vi "REPORT_AUDIT_rows_style_pdf.vi"(11 "REPORT_AUDIT_all_info":T1) -> (3 "Row  [ ]":T3)   [LabVIEW 2020]
uses:
  <vilib>/Exaprom PDF/Controls/Table Controls/Table Appearance and Font Row [ ].ctl
  <vilib>/Exaprom PDF/Controls/Table Controls/One Row Appearance.ctl
  <vilib>/Exaprom PDF/Controls/Table Controls/Row from to.ctl
  <vilib>/Exaprom PDF/Controls/Table Controls/Cell, Alignment, LS and Font - hide Vmerge.ctl
  <vilib>/Exaprom PDF/Controls/Table Controls/Cell Type, Alignment and LS.ctl
  <vilib>/Exaprom PDF/Controls/Table Controls/Cell Alignment 20px.ctl
  <vilib>/Exaprom PDF/Controls/Table Controls/Text vertical arrangement.ctl
  <vilib>/Exaprom PDF/Controls/Text Controls/Line spacing.ctl
  <vilib>/Exaprom PDF/Controls/Table Controls/Cell Appearance.ctl
  <vilib>/Exaprom PDF/Controls/Table Controls/Cell Border 20 px.ctl
  <vilib>/Exaprom PDF/Controls/Table Controls/Merge Horizontal.ctl
  <vilib>/Exaprom PDF/Controls/Table Controls/Merge Vertical.ctl
  <vilib>/Exaprom PDF/Controls/Font Controls/Font complete cluster.ctl
  <vilib>/Exaprom PDF/Controls/Font Controls/Font size.ctl
  <vilib>/Exaprom PDF/Controls/Font Controls/Font color.ctl
  <vilib>/Exaprom PDF/Controls/Font Controls/Type and encoding.ctl
  <vilib>/Exaprom PDF/Controls/Text Controls/Unicode/Type and run direction.ctl
  typedef/REPORT_AUDIT_all_info.ctl
  GEAR/typedef/REPORT_GEAR_statuses.ctl
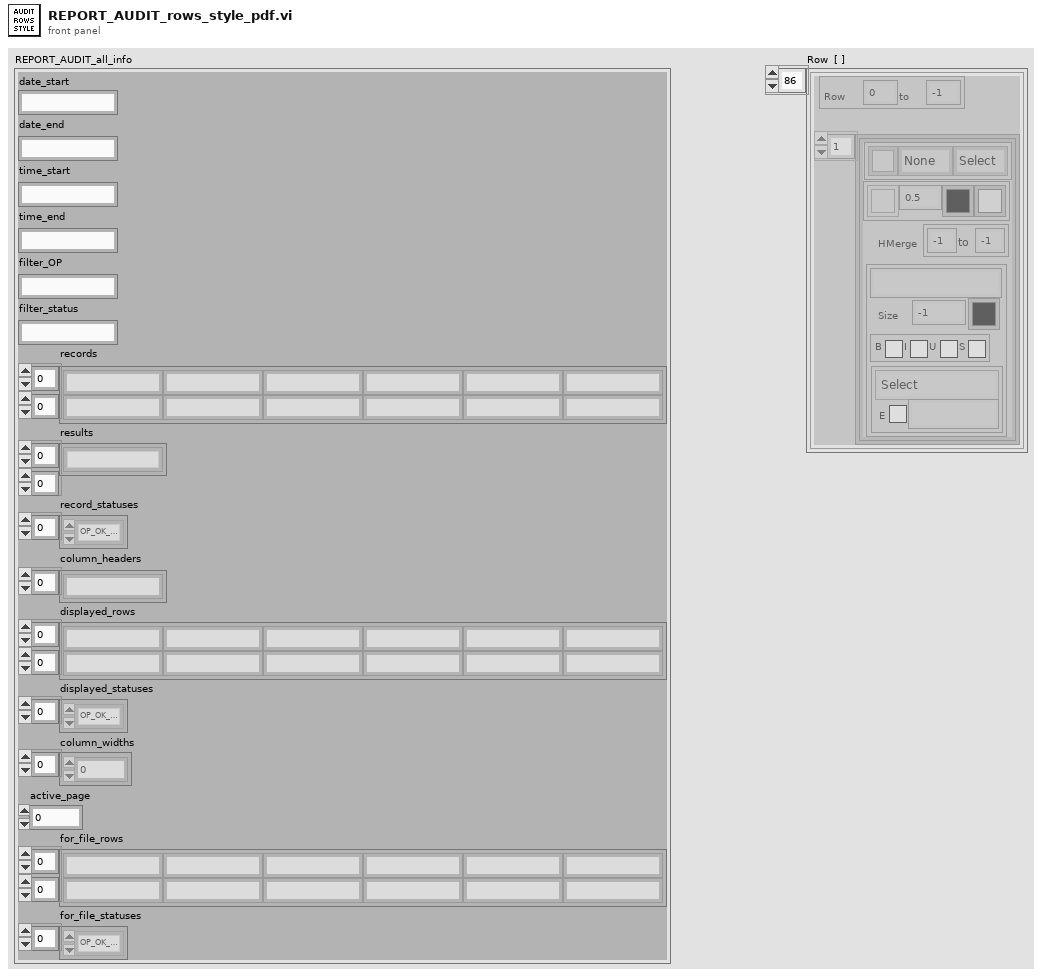
[diagram p1: front panel]
types:
  T1 = typedef "REPORT_AUDIT_all_info.ctl" = cluster{"date_start":string, "date_end":string, "time_start":string, "time_end":string, "filter_OP":string, "filter_status":string, "records":string[][], "results":string[][], "record_statuses":T2[], "column_headers":string[], "displayed_rows":string[][], "displayed_statuses":T2[], "column_widths":i16[], "active_page":i32, "for_file_rows":string[][], "for_file_statuses":T2[]}
  T2 = typedef "REPORT_GEAR_statuses.ctl" = enum16{"OP_OK_hide", "OP_OK_show", "OP_NOK_hide", "OP_NOK_show", "OP_interrupted_hide", "OP_interrupted_show", "OP_in_operation_hide", "OP_in_operation_show", "OP_unexpected_hide", "OP_unexpected_show", "RE_REAL_OK", "RE_REAL_NOK", "RE_STRING", "RE_sub_header", "RE_no_data", "RE_unexpected", "BA_sub_header", "BA_data", "BA_no_data"}
  T3 = typedef "Table Appearance and Font Row [ ].ctl" = T4[]
  T4 = typedef "One Row Appearance.ctl" = cluster{"Row":T5, "Cell [ ]":T6[]}
  T5 = typedef "Row from to.ctl" = cluster{"From #":i16, "to #":i16}
  T6 = typedef "Cell, Alignment, LS and Font - hide Vmerge.ctl" = cluster{"Text":T7, "Cell Appearance":T11, "HMerge":T13, "VMerge":T14, "Font":T15}
  T7 = typedef "Cell Type, Alignment and LS.ctl" = cluster{"Cell Alignment":T8, "Text rotation":T9, "Line spacing":T10}
  T8 = typedef "Cell Alignment 20px.ctl" = u16
  T9 = typedef "Text vertical arrangement.ctl" = enum16{"None", "Clockwise", "Counterclockwise"}
  T10 = typedef "Line spacing.ctl" = enum16{"Select", "1.0", "1.5", "2.0"}
  T11 = typedef "Cell Appearance.ctl" = cluster{"Border":T12, "Thickness":sgl, "Color":u32, "BG":u32}
  T12 = typedef "Cell Border 20 px.ctl" = u16
  T13 = typedef "Merge Horizontal.ctl" = cluster{"From":i8, "to":i8}
  T14 = typedef "Merge Vertical.ctl" = cluster{"From":i8, "to":i8}
  T15 = typedef "Font complete cluster.ctl" = cluster{"Name":string, "Size":T16, "Color":T17, "Style":cluster{"Bold":bool, "Italic":bool, "Underline":bool, "Strikeout":bool}, "Type":T18}
  T16 = typedef "Font size.ctl" = sgl
  T17 = typedef "Font color.ctl" = u32
  T18 = typedef "Type and encoding.ctl" = cluster{"Type&direction":T19, "Embedded":bool, "Encoding":string}
  T19 = typedef "Type and run direction.ctl" = enum16{"Select", "ASCII", "UTF-16", "UTF-16 (default)", "UTF-16 (LTR)", "UTF-16 (RTL)"}
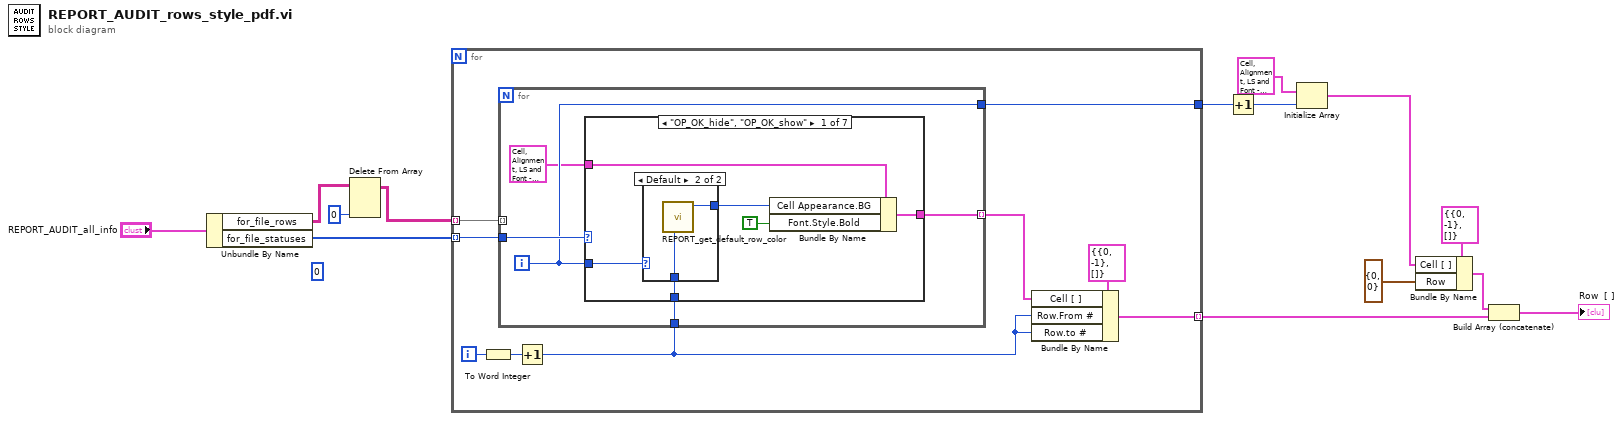
[diagram p0: block diagram]
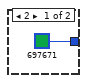
[diagram p2: hidden frame]
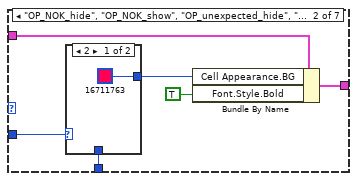
[diagram p3: hidden frame]
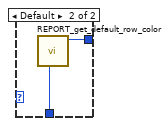
[diagram p4: hidden frame]
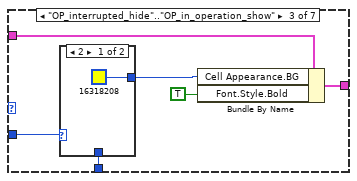
[diagram p5: hidden frame]
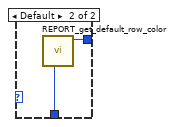
[diagram p6: hidden frame]
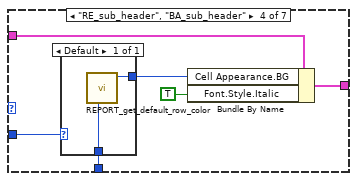
[diagram p7: hidden frame]
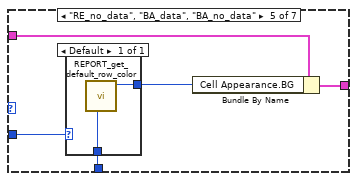
[diagram p8: hidden frame]
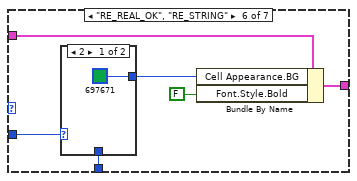
[diagram p9: hidden frame]
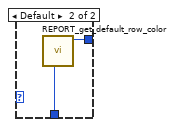
[diagram p10: hidden frame]
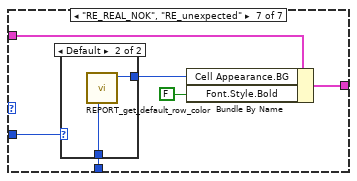
[diagram p11: hidden frame]
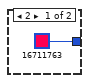
[diagram p12: hidden frame]
diagram:
  (unwired) 0
  n1 = Unbundle By Name("REPORT_AUDIT_all_info") -> ("for_file_rows"=w4:string[][], "for_file_statuses"=w1:T2[])
  n2 = Delete From Array(array=w4, index (col)=0) -> (array with subset deleted=w2:string[][])  [unwired: 2 in, 1 out]
  n3 = for {
    tunnel: w2 -> [w19] mode=indexing
    tunnel: w1 -> [w18] mode=indexing
    tunnel: [w22] -> w12 mode=indexing
    tunnel: [w15] -> w6
    i -> [w21]
    n4 = To Word Integer(number=w21) -> (16bit integer=w20:i16)
    n5 = Increment(x=w20) -> (x+1=w16:i16)
    n6 = for {
      tunnel: w19 -> [_] mode=indexing
      tunnel: w18 -> [w28]
      tunnel: [w27] -> w17 mode=indexing
      tunnel: w16 -> [w24]
      tunnel: [w26] -> w15
      i -> [w26]
      n7 = case shown="\"OP_OK_hide\", \"OP_OK_show\"" w28 {
        tunnel: T6 {"Text"={"Cell Alignment"=0, "Text rotation"=enum."None", "Line spacing"=enum."Select"}, "Cell Appearance"={"Border"=5, "Thickness"=0.5, "Color"=0, "BG"=16448250}, "HMerge"={"From"=-1, "to"=-1}, "VMerge"={"From"=-1, "to"=-1}, "Font"={"Name"="Consolas", "Size"=10.0, "Color"=0, "Style"={"Bold"=FALSE, "Italic"=FALSE, "Underline"=FALSE, "Strikeout"=FALSE}, "Type"={"Type&direction"=enum."ASCII", "Embedded"=FALSE, "Encoding"="CP855"}}} ("Cell, Alignment, LS and Font") -> [w34 w41 w50 w59 w66 w73 w82]
        tunnel: [w31 w40 w47 w58 w67 w74 w83] -> w27
        tunnel: w26 -> [w30 w39 w49 w56 w65 w72 w81]
        tunnel: w24 -> [w29 w38 w48 w57 w64 w71 w80]
        frame "OP_OK_hide", "OP_OK_show" {
          n8 = case shown="Default" w30 {
            tunnel: [u32 697671 w37] -> w32
            tunnel: w29 -> [_ w36]
            frame 2 {
            }
            frame Default {
              n9 = call "REPORT_get_default_row_color.vi"("row"=w36) -> ("color"=w37:u32)  [unwired: 10 in]
            }
          }
          n10 = Bundle By Name(cluster=w34, "Cell Appearance.BG"=w32, "Font.Style.Bold"=TRUE ("Active Cell:Cell Font:Bold")) -> (w31:T6)
        }
        frame "OP_NOK_hide", "OP_NOK_show", "OP_unexpected_hide", "OP_unexpected_show" {
          n11 = case shown="2" w39 {
            tunnel: [u32 16711763 w46] -> w42
            tunnel: w38 -> [_ w45]
            frame 2 {
            }
            frame Default {
              n12 = call "REPORT_get_default_row_color.vi"("row"=w45) -> ("color"=w46:u32)  [unwired: 10 in]
            }
          }
          n13 = Bundle By Name(cluster=w41, "Cell Appearance.BG"=w42, "Font.Style.Bold"=TRUE ("Active Cell:Cell Font:Bold")) -> (w40:T6)
        }
        frame "OP_interrupted_hide".."OP_in_operation_show" {
          n14 = case shown="2" w49 {
            tunnel: [u32 16318208 w55] -> w52
            tunnel: w48 -> [_ w54]
            frame 2 {
            }
            frame Default {
              n15 = call "REPORT_get_default_row_color.vi"("row"=w54) -> ("color"=w55:u32)  [unwired: 10 in]
            }
          }
          n16 = Bundle By Name(cluster=w50, "Cell Appearance.BG"=w52, "Font.Style.Bold"=TRUE ("Active Cell:Cell Font:Bold")) -> (w47:T6)
        }
        frame "RE_sub_header", "BA_sub_header" {
          n17 = case shown="Default" w56 {
            tunnel: [w63] -> w61
            tunnel: w57 -> [w62]
            frame Default {
              n18 = call "REPORT_get_default_row_color.vi"("row"=w62) -> ("color"=w63:u32)  [unwired: 10 in]
            }
          }
          n19 = Bundle By Name(cluster=w59, "Cell Appearance.BG"=w61, "Font.Style.Italic"=TRUE ("Active Cell:Cell Font:Bold")) -> (w58:T6)
        }
        frame "RE_no_data", "BA_data", "BA_no_data" {
          n20 = case shown="Default" w65 {
            tunnel: [w70] -> w68
            tunnel: w64 -> [w69]
            frame Default {
              n21 = call "REPORT_get_default_row_color.vi"("row"=w69) -> ("color"=w70:u32)  [unwired: 10 in]
            }
          }
          n22 = Bundle By Name(cluster=w66, "Cell Appearance.BG"=w68) -> (w67:T6)
        }
        frame "RE_REAL_OK", "RE_STRING" {
          n23 = case shown="2" w72 {
            tunnel: [u32 697671 w79] -> w76
            tunnel: w71 -> [_ w78]
            frame 2 {
            }
            frame Default {
              n24 = call "REPORT_get_default_row_color.vi"("row"=w78) -> ("color"=w79:u32)  [unwired: 10 in]
            }
          }
          n25 = Bundle By Name(cluster=w73, "Cell Appearance.BG"=w76, "Font.Style.Bold"=FALSE ("Active Cell:Cell Font:Bold")) -> (w74:T6)
        }
        frame "RE_REAL_NOK", "RE_unexpected" {
          n26 = case shown="Default" w81 {
            tunnel: [u32 16711763 w88] -> w85
            tunnel: w80 -> [_ w87]
            frame 2 {
            }
            frame Default {
              n27 = call "REPORT_get_default_row_color.vi"("row"=w87) -> ("color"=w88:u32)  [unwired: 10 in]
            }
          }
          n28 = Bundle By Name(cluster=w82, "Cell Appearance.BG"=w85, "Font.Style.Bold"=FALSE ("Active Cell:Cell Font:Bold")) -> (w83:T6)
        }
      }
    }
    n29 = Bundle By Name(cluster=T4 {"Row"={"From #"=0, "to #"=-1}, "Cell [ ]"=[]} ("Row Appearance and Font  [ ]"), "Cell [ ]"=w17, "Row.From #"=w16, "Row.to #"=w16) -> (w22:T4)
  }
  n30 = Increment(x=w6) -> (x+1=w5:i32)
  n31 = Initialize Array(T6 {"Text"={"Cell Alignment"=0, "Text rotation"=enum."None", "Line spacing"=enum."Select"}, "Cell Appearance"={"Border"=5, "Thickness"=1.5, "Color"=16777228, "BG"=16448250}, "HMerge"={"From"=-1, "to"=-1}, "VMerge"={"From"=-1, "to"=-1}, "Font"={"Name"="Consolas", "Size"=10.0, "Color"=16777228, "Style"={"Bold"=TRUE, "Italic"=FALSE, "Underline"=FALSE, "Strikeout"=FALSE}, "Type"={"Type&direction"=enum."ASCII", "Embedded"=FALSE, "Encoding"="CP855"}}} ("Cell, Alignment, LS and Font"), w5) -> (w8:T6[])
  n32 = Bundle By Name(cluster=T4 {"Row"={"From #"=0, "to #"=-1}, "Cell [ ]"=[]} ("Row Appearance and Font  [ ]"), "Cell [ ]"=w8, "Row"=T5 {"From #"=0, "to #"=0}) -> (w10:T4)
  n33 = Build Array (concatenate)(w10, w12) -> (→"Row  [ ]":T4[])
